vi "Close Shutters.vi"(8 "error in (no error)":errorcluster) -> (0 "error out (no error)":errorcluster)   [LabVIEW 2020]
uses:
  Typedefs/PMT control functions.ctl
  Typedefs/Shutter Function Enum.ctl
  Global Variables/General Globals.vi
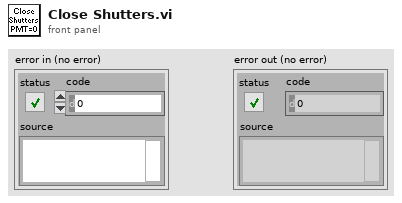
[diagram p1: front panel]
types:
  T1 = typedef "Shutter Function Enum.ctl" = enum16{"Open Shutter", "Close Shutter"}
  T2 = typedef "PMT control functions.ctl" = enum16{"Set PMTs from UI", "Reset PMTs"}
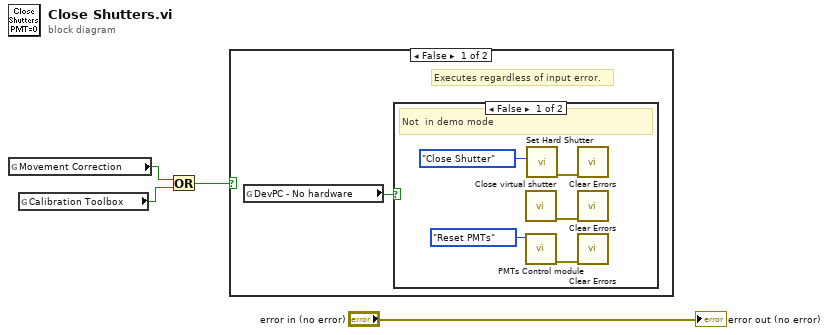
[diagram p0: block diagram]
diagram:
  n1 = global read "General Globals.vi" "Movement Correction"() -> (w3:bool)
  n2 = global read "General Globals.vi" "Calibration Toolbox"() -> (w2:bool)
  n3 = Or(x=w3, y=w2) -> (x .or. y?=w1:bool)
  n4 = case shown="False" w1 {
    frame False {
      # "Executes regardless of input error."
      n5 = global read "General Globals.vi" "DevPC - No hardware"() -> (w5:bool)
      n6 = case shown="False" w5 {
        frame False {
          # "Not  in demo mode"
          n7 = call "Close virtual shutter.vi"() -> ("error out"=w8:errorcluster)  [unwired: 11 in]
          n8 = call "PMTs Control module.vi"("Function"=PMT_control_functions."Reset PMTs") -> ("Error Out"=w9:errorcluster)  [unwired: 10 in]
          n9 = call "Set Hard Shutter.vi"("Shutter Function"=Shutter_Function_Enum."Close Shutter") -> ("Error Out"=w6:errorcluster)  [unwired: 10 in]
          n10 = call <vilib>:"Clear Errors.vi"("error in (no error)"=w6) -> ()  [unwired: 5 in, 2 out]
          n11 = call <vilib>:"Clear Errors.vi"("error in (no error)"=w8) -> ()  [unwired: 5 in, 2 out]
          n12 = call <vilib>:"Clear Errors.vi"("error in (no error)"=w9) -> ()  [unwired: 5 in, 2 out]
        }
        frame True {
          # "Demo mode"
        }
      }
    }
    frame True {
    }
  }
  "error out (no error)" <- "error in (no error)"
